vi "deep cluster.vi"(10 "Cluster":T1={"a"=0.0, "Cluster"={"a"=1.0, "Cluster"={"a"=2.0, "Cluster"={"a"=3.0, "Cluster"={"a"=4.0, "Cluster"={"a"=5.0, "Cluster"={"a"=6.0, "Cluster"={"a"=7.0, "Cluster"={"a"=8.0, "Cluster"={"a"=9.0, "Cluster"={"a"=10.0}}}}}}}}}}}) -> (2 "Cluster 2":T1={"a"=0.0, "Cluster"={"a"=1.0, "Cluster"={"a"=2.0, "Cluster"={"a"=3.0, "Cluster"={"a"=4.0, "Cluster"={"a"=5.0, "Cluster"={"a"=6.0, "Cluster"={"a"=7.0, "Cluster"={"a"=8.0, "Cluster"={"a"=9.0, "Cluster"={"a"=10.0}}}}}}}}}}})   [LabVIEW 2012]
panel:
  in  "a":dbl
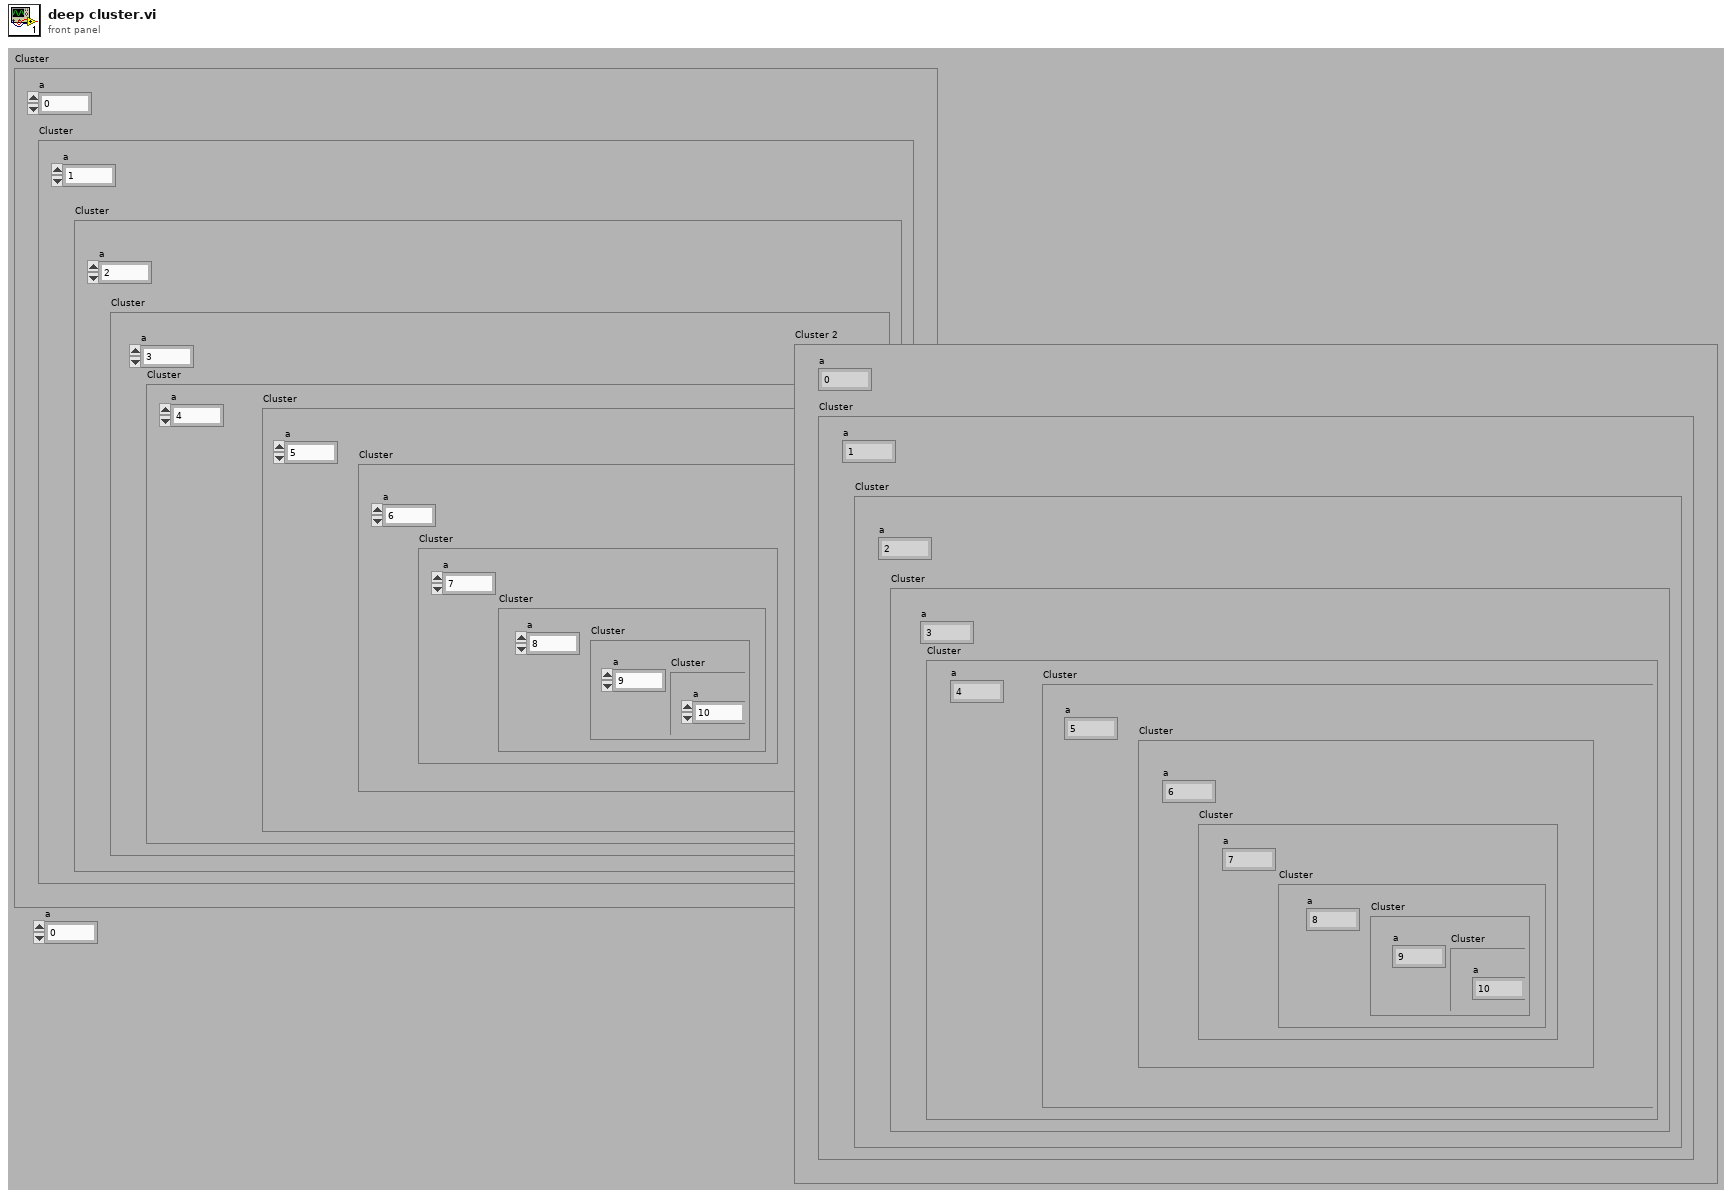
[diagram p1: front panel]
types:
  T1 = cluster{"a":dbl, "Cluster":cluster{"a":dbl, "Cluster":cluster{"a":dbl, "Cluster":cluster{"a":dbl, "Cluster":cluster{"a":dbl, "Cluster":cluster{"a":dbl, "Cluster":cluster{"a":dbl, "Cluster":cluster{"a":dbl, "Cluster":cluster{"a":dbl, "Cluster":cluster{"a":dbl, "Cluster":cluster{"a":dbl}}}}}}}}}}}
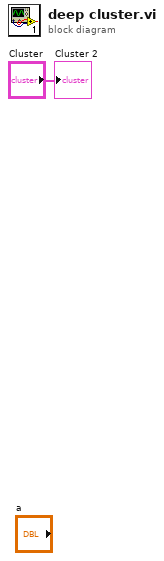
[diagram p0: block diagram]
diagram:
  "Cluster 2" <- "Cluster"
